vi "Linear Interpolation for Monotonic arrays.vi"(1 "Desired X":dbl, 2 "Y Array":dbl[](array[numeric]), 3 "X Array":dbl[](array[numeric])) -> (0 "Calculated Y":dbl)   [LabVIEW 2022 SP3]
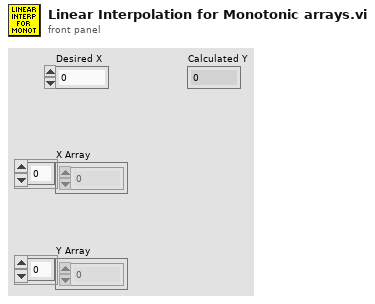
[diagram p1: front panel]
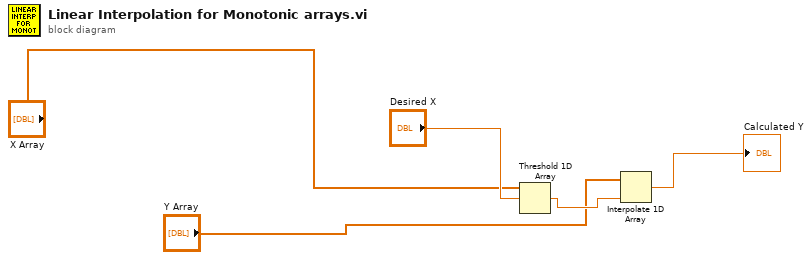
[diagram p0: block diagram]
diagram:
  n1 = Threshold 1D Array(2:"Desired X", 3:"X Array") -> (0:w3:dbl)  [unwired: 1 in]
  n2 = Interpolate 1D Array(1:w3, 2:"Y Array") -> (0:→"Calculated Y":dbl)
